vi "fbp.vi"(9 "Keep pixels?":bool, 10 "Image Properties":T4, 11 "Backproject Input":T1) -> (1 "Projection Pixels":T2(array[cluster]), 2 "Projections":T3[](array[typedef]), 3 "Output":sgl[](array[numeric]))   [LabVIEW 2013]
uses:
  tags_cluster.ctl
  bp_work_unit.ctl
  backproject_input.ctl
  pixels_for_proj.ctl
panel:
  out "Normalisation":i32[](array[numeric])
  out "Current summing work unit #":i32
  out "destroyed queue name":string
  out "Selector":dbl
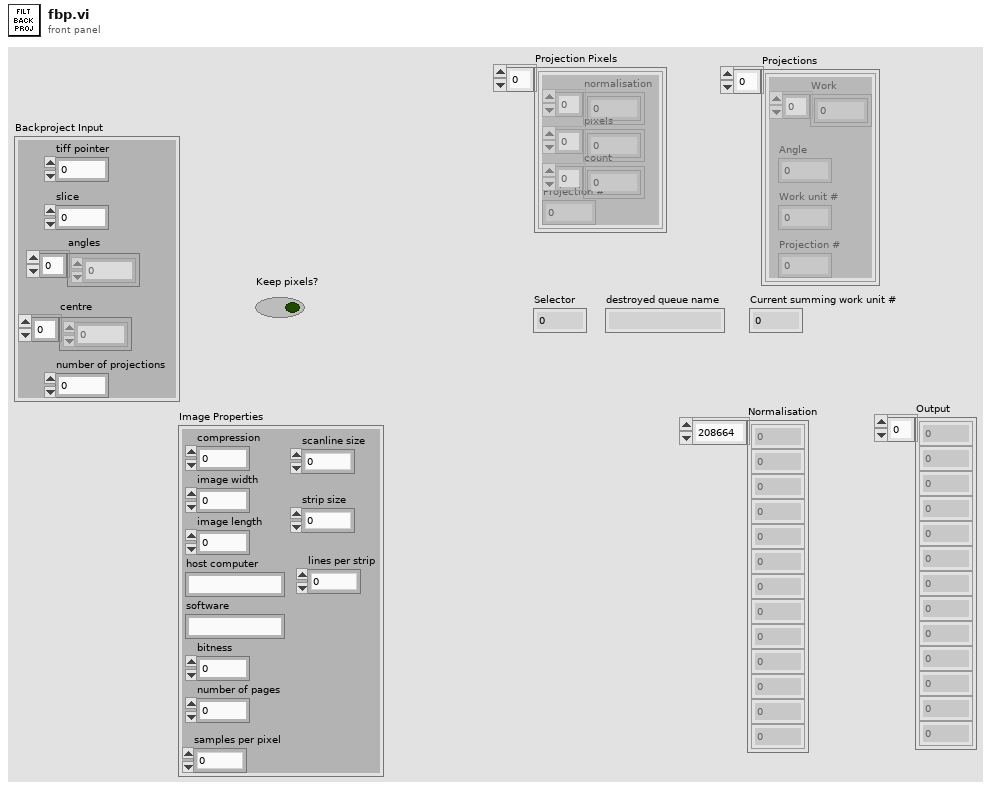
[diagram p1: front panel]
types:
  T1 = typedef "backproject_input.ctl" = cluster{"tiff pointer":i64, "slice":u32, "angles":dbl[], "centre":i32[], "number of projections":u32}
  T2 = cluster{"normalisation":i32[], "pixels":i32[], "count":i32[], "Projection #":i32}[]
  T3 = typedef "bp_work_unit.ctl" = cluster{"Work":u8[], "Angle":dbl, "Work unit #":i32, "Projection #":i32}
  T4 = typedef "tags_cluster.ctl" = cluster{"compression":i32, "image width":i32, "image length":i32, "host computer":string, "software":string, "bitness":i32, "number of pages":i32, "samples per pixel":i32, "scanline size":i32, "strip size":i32, "lines per strip":i32}
  T5 = typedef "pixels_for_proj.ctl" = cluster{"normalisation":i32[], "pixels":i32[], "count":i32[], "Projection #":i32}
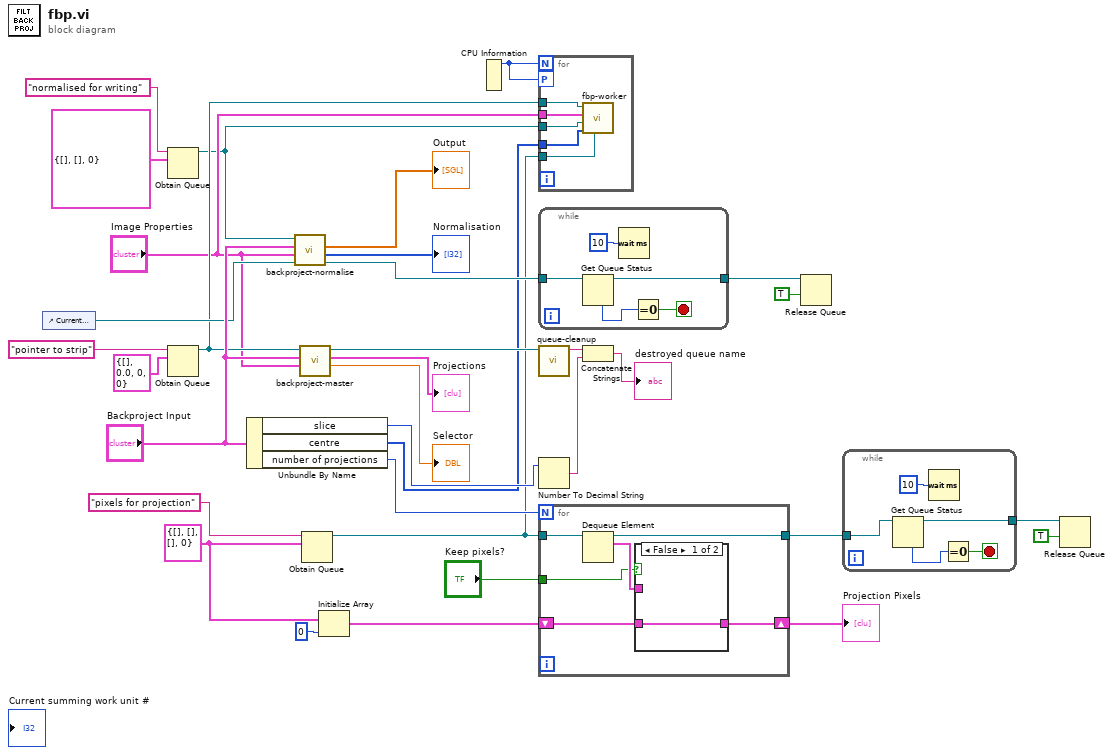
[diagram p0: block diagram]
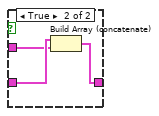
[diagram p2: hidden frame]
diagram:
  w24 = T5 {"normalisation"=[], "pixels"=[], "count"=[], "Projection #"=0}
  n1 = control-ref of="Current summing work unit #"() -> (w14:refnum<vi>)
  n2 = Obtain Queue(name (unnamed)="normalised for writing", element data type=cluster{sgl[], i32[], i32} {[], [], 0}) -> (queue out=w2:refnum<queue>)  [unwired: 3 in, 2 out]
  n3 = Obtain Queue(name (unnamed)="pointer to strip", element data type=T3 {"Work"=[], "Angle"=0.0, "Work unit #"=0, "Projection #"=0} ("backproject work unit")) -> (queue out=w6:refnum<queue>)  [unwired: 3 in, 2 out]
  n4 = Unbundle By Name("Backproject Input") -> ("slice"=w18:u32, "centre"=w3:i32[], "number of projections"=w16:u32)
  n5 = call "backproject-normalise.vi"("Ctl Refnum"=w14, "Image Properties"="Image Properties", "Backproject Input"="Backproject Input", "Queue in"=w2) -> ("queue out"=w8:refnum<queue>, "Normalisation"=→"Normalisation":i32[], "Array"=→"Output":sgl[])  [unwired: 4 in, 1 out]
  n6 = call "backproject-master.vi"("Image Properties"="Image Properties", "Backproject Input"="Backproject Input", "Queue in"=w6) -> ("Selector"=→"Selector":dbl, "Projections"=→"Projections":T3[], "Queue out"=w20:refnum<queue>)  [unwired: 6 in]
  n7 = Obtain Queue(name (unnamed)="pixels for projection", element data type=w24) -> (queue out=w4:refnum<queue>)  [unwired: 3 in, 2 out]
  n8 = Initialize Array(w24, 0 ("dimension size")) -> (w22:T5[])
  n9 = CPU Information() -> (4:w1:i32)  [unwired: 3 out]
  n10 = for {
    N: w1 -> [_]
    tunnel: w6 -> [w39]
    tunnel: "Image Properties" -> [w38]
    tunnel: w4 -> [w37]
    tunnel: w3 -> [w36]
    tunnel: w2 -> [w35]
    workers-P: w1 -> [_]
    n11 = call "fbp-worker.vi"("pixels for projections"=w37, "Centre"=w36, "Write queue"=w35, "Image Properties"=w38, "Work queue in"=w39) -> ()  [unwired: 4 in, 3 out]
  }
  n12 = while {
    tunnel: [w42] -> w9
    tunnel: w8 -> [w40]
    stop <- w43 stop-if-true
    n13 = Get Queue Status(queue=w40) -> (queue out=w42:refnum<queue>, # elements in queue=w44:i32)  [unwired: 2 in, 6 out]
    n14 = Wait (ms)(milliseconds to wait=u32 10) -> ()  [unwired: 1 out]
    n15 = Equal To 0?(x=w44) -> (x = 0?=w43:bool)
  }
  n16 = call "queue-cleanup.vi"("Queue in"=w20) -> ("queue name"=w27:string)  [unwired: 10 in]
  n17 = Number To Decimal String(number=w18) -> (decimal integer string=w26:string)  [unwired: 1 in]
  n18 = for {
    N: w16 -> [_]
    tunnel: w4 -> [w50]
    shift-right: [w48] -> w21
    shift-left: w22 -> [w49]
    tunnel: [w46] -> w11
    tunnel: "Keep pixels?" -> [w45]
    n19 = Dequeue Element(queue=w50) -> (queue out=w46:refnum<queue>, element=w47:T5)  [unwired: 2 in, 2 out]
    n20 = case shown="False" w45 {
      tunnel: w49 -> [w51 w54]
      tunnel: [w51 w53] -> w48
      tunnel: w47 -> [_ w52]
      frame False {
      }
      frame True {
        n21 = Build Array (concatenate)(w54, w52) -> (w53:T5[])
      }
    }
  }
  "Projection Pixels" <- w21
  n22 = Concatenate Strings(w27, w26) -> (→"destroyed queue name":string)
  n23 = Release Queue(queue=w9, force destroy? (F)=TRUE) -> ()  [unwired: 1 in, 3 out]
  n24 = while {
    tunnel: [w57] -> w13
    tunnel: w11 -> [w55]
    stop <- w58 stop-if-true
    n25 = Get Queue Status(queue=w55) -> (queue out=w57:refnum<queue>, # elements in queue=w59:i32)  [unwired: 2 in, 6 out]
    n26 = Wait (ms)(milliseconds to wait=u32 10) -> ()  [unwired: 1 out]
    n27 = Equal To 0?(x=w59) -> (x = 0?=w58:bool)
  }
  n28 = Release Queue(queue=w13, force destroy? (F)=TRUE) -> ()  [unwired: 1 in, 3 out]
